vi "Periodic Tasks.vi"(8 "error in":errorcluster) -> ()   [LabVIEW 2019]
doc: "This VI runs in parallel to other tasks. It can contain as many user-defined periodic loops as you need. These can carry out PID or other sorts of timed response."
uses:
  <vilib>/Rock Robotics/WPI/Utilities/WPI_GetSetVariantRefNum.vi
  Robot Global Data.vi
  Secret_Control_Library_Protected/TIME_GET.vi
  <vilib>/addons/control/pid/pid.llb/PID (DBL).vi
  <vilib>/Rock Robotics/Network Tables/NT Write Numeric Array.vi
  <vilib>/Rock Robotics/Network Tables/NT Write Number.vi
  <vilib>/Rock Robotics/Network Tables/NT Write Boolean.vi
  Secret_Control_Library_Protected/Secret_Control_Library_Protected.lvlib
  <vilib>/addons/control/pid/NI_PID_pid.lvlib
  <vilib>/Rock Robotics/WPI/ThirdParty/JAS_Junk/TrajLib/Trajectory_Library.lvlib
panel:
  in  "Speed PID":T1={"proportional gain (Kc)"=0.6, "integral time (Ti, min)"=0.015, "derivative time (Td, min)"=0.0} {"derivative time (Td, min)" format="%.3f"; "integral time (Ti, min)" format="%.3f"; "proportional gain (Kc)" format="%.3f"}
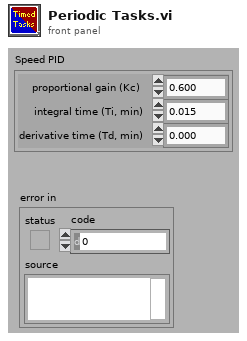
[diagram p1: front panel]
types:
  T1 = cluster{"proportional gain (Kc)":dbl, "integral time (Ti, min)":dbl, "derivative time (Td, min)":dbl}
  T2 = typedef "WPI_EncoderDevRef.ctl" = cluster{"DevStatus":errorcluster, "EncoderIndex":T3, "CounterIndex":T4, "DistancePerCount":dbl, "Decoding Type":T5}
  T3 = typedef "FPGA_EncoderIdx.ctl" = enum8{"Enc 0", "Enc 1", "Enc 2", "Enc 3", "Enc 4", "Enc 5", "Enc 6", "Enc 7", "Invalid"}
  T4 = typedef "FPGA_CounterCtrSystemIndex.ctl" = enum8{"Ctr 0", "Ctr 1", "Ctr 2", "Ctr 3", "Ctr 4", "Ctr 5", "Ctr 6", "Ctr 7", "Invalid"}
  T5 = typedef "WPI_EncoderType.ctl" = enum16{"1x", "2x", "4x"}
  T6 = typedef "WPI_GyroDevRef.ctl" = cluster{"DevStatus":errorcluster, "Analog Channel":T7, "Gain (VoltsPerDegree/Second)":dbl, "Gyro Type":enum16{"Analog", "XRS450"}, "Handle":i32, "SPI Bus":T8, "Device Found":bool, "Sample Rate":dbl, "Calibrate On Open":bool, "Offset":dbl}
  T7 = typedef "FPGA_AIChannel.ctl" = enum8{"AI 0", "AI 1", "AI 2", "AI 3", "AI MXP 0", "AI MXP 1", "AI MXP 2", "AI MXP 3", "Invalid"}
  T8 = typedef "spi_bus.ctl" = enum16{"SPI On-Board, CS0", "SPI On-Board, CS1", "SPI On-Board, CS2", "SPI On-Board, CS3", "SPI MXP", "Invalid"}
  T9 = typedef "WPI_RobotDriveDevRef.ctl" = cluster{"DevStatus":errorcluster, "Motors[]":T10[], "Square Inputs":bool, "Max Output":dbl}
  T10 = typedef "WPI_MotorControlDeviceRef.ctl" = cluster{"DeviceStatus":errorcluster, "Type":T11, "PWM":cluster{"PWM Channel":T12, "DeadBand":T13}, "CAN":cluster{"Device Number":u8, "SetOutput VI Ref":variant, "GetOutput VI Ref":variant, "Enable VI Ref":variant, "Disable VI Ref":variant, "Data":variant}, "Invert":bool, "DIO PWM":cluster{"PWM \"Enable\" Channel":T12, "DIOChannel":T14, "PWM Rate":dbl}}
  T11 = typedef "WPI_MotorControlType.ctl" = enum16{"PWM", "CAN", "DIO PWM"}
  T12 = typedef "FPGA_DIOPWMChannel.ctl" = enum8{"PWM 0", "PWM 1", "PWM 2", "PWM 3", "PWM 4", "PWM 5", "PWM 6", "PWM 7", "PWM 8", "PWM 9", "PWM MXP 0", "PWM MXP 1", "PWM MXP 2", "PWM MXP 3", "PWM MXP 4", "PWM MXP 5", "PWM MXP 6", "PWM MXP 7", "PWM MXP 8", "PWM MXP 9", "Invalid"}
  T13 = typedef "WPI_PWMDeadband.ctl" = cluster{"Name":string, "maxPositivePwm":i32, "minPositivePwm":i32, "centerPwm":i32, "maxNegativePwm":i32, "minNegativePwm":i32, "angularRange":u16}
  T14 = typedef "FPGA_DIOChannel.ctl" = enum8{"DIO 0", "DIO 1", "DIO 2", "DIO 3", "DIO 4", "DIO 5", "DIO 6", "DIO 7", "DIO 8", "DIO 9", "DIO MXP 0", "DIO MXP 1", "DIO MXP 2", "DIO MXP 3", "DIO MXP 4", "DIO MXP 5", "DIO MXP 6", "DIO MXP 7", "DIO MXP 8", "DIO MXP 9", "DIO MXP 10", "DIO MXP 11", "DIO MXP 12", "DIO MXP 13", "DIO MXP 14", "DIO MXP 15", "SPI Port CS1", "SPI Port CS2", "SPI Port CS3", "SPI Port MISO", "SPI Port MOSI", "Invalid"}
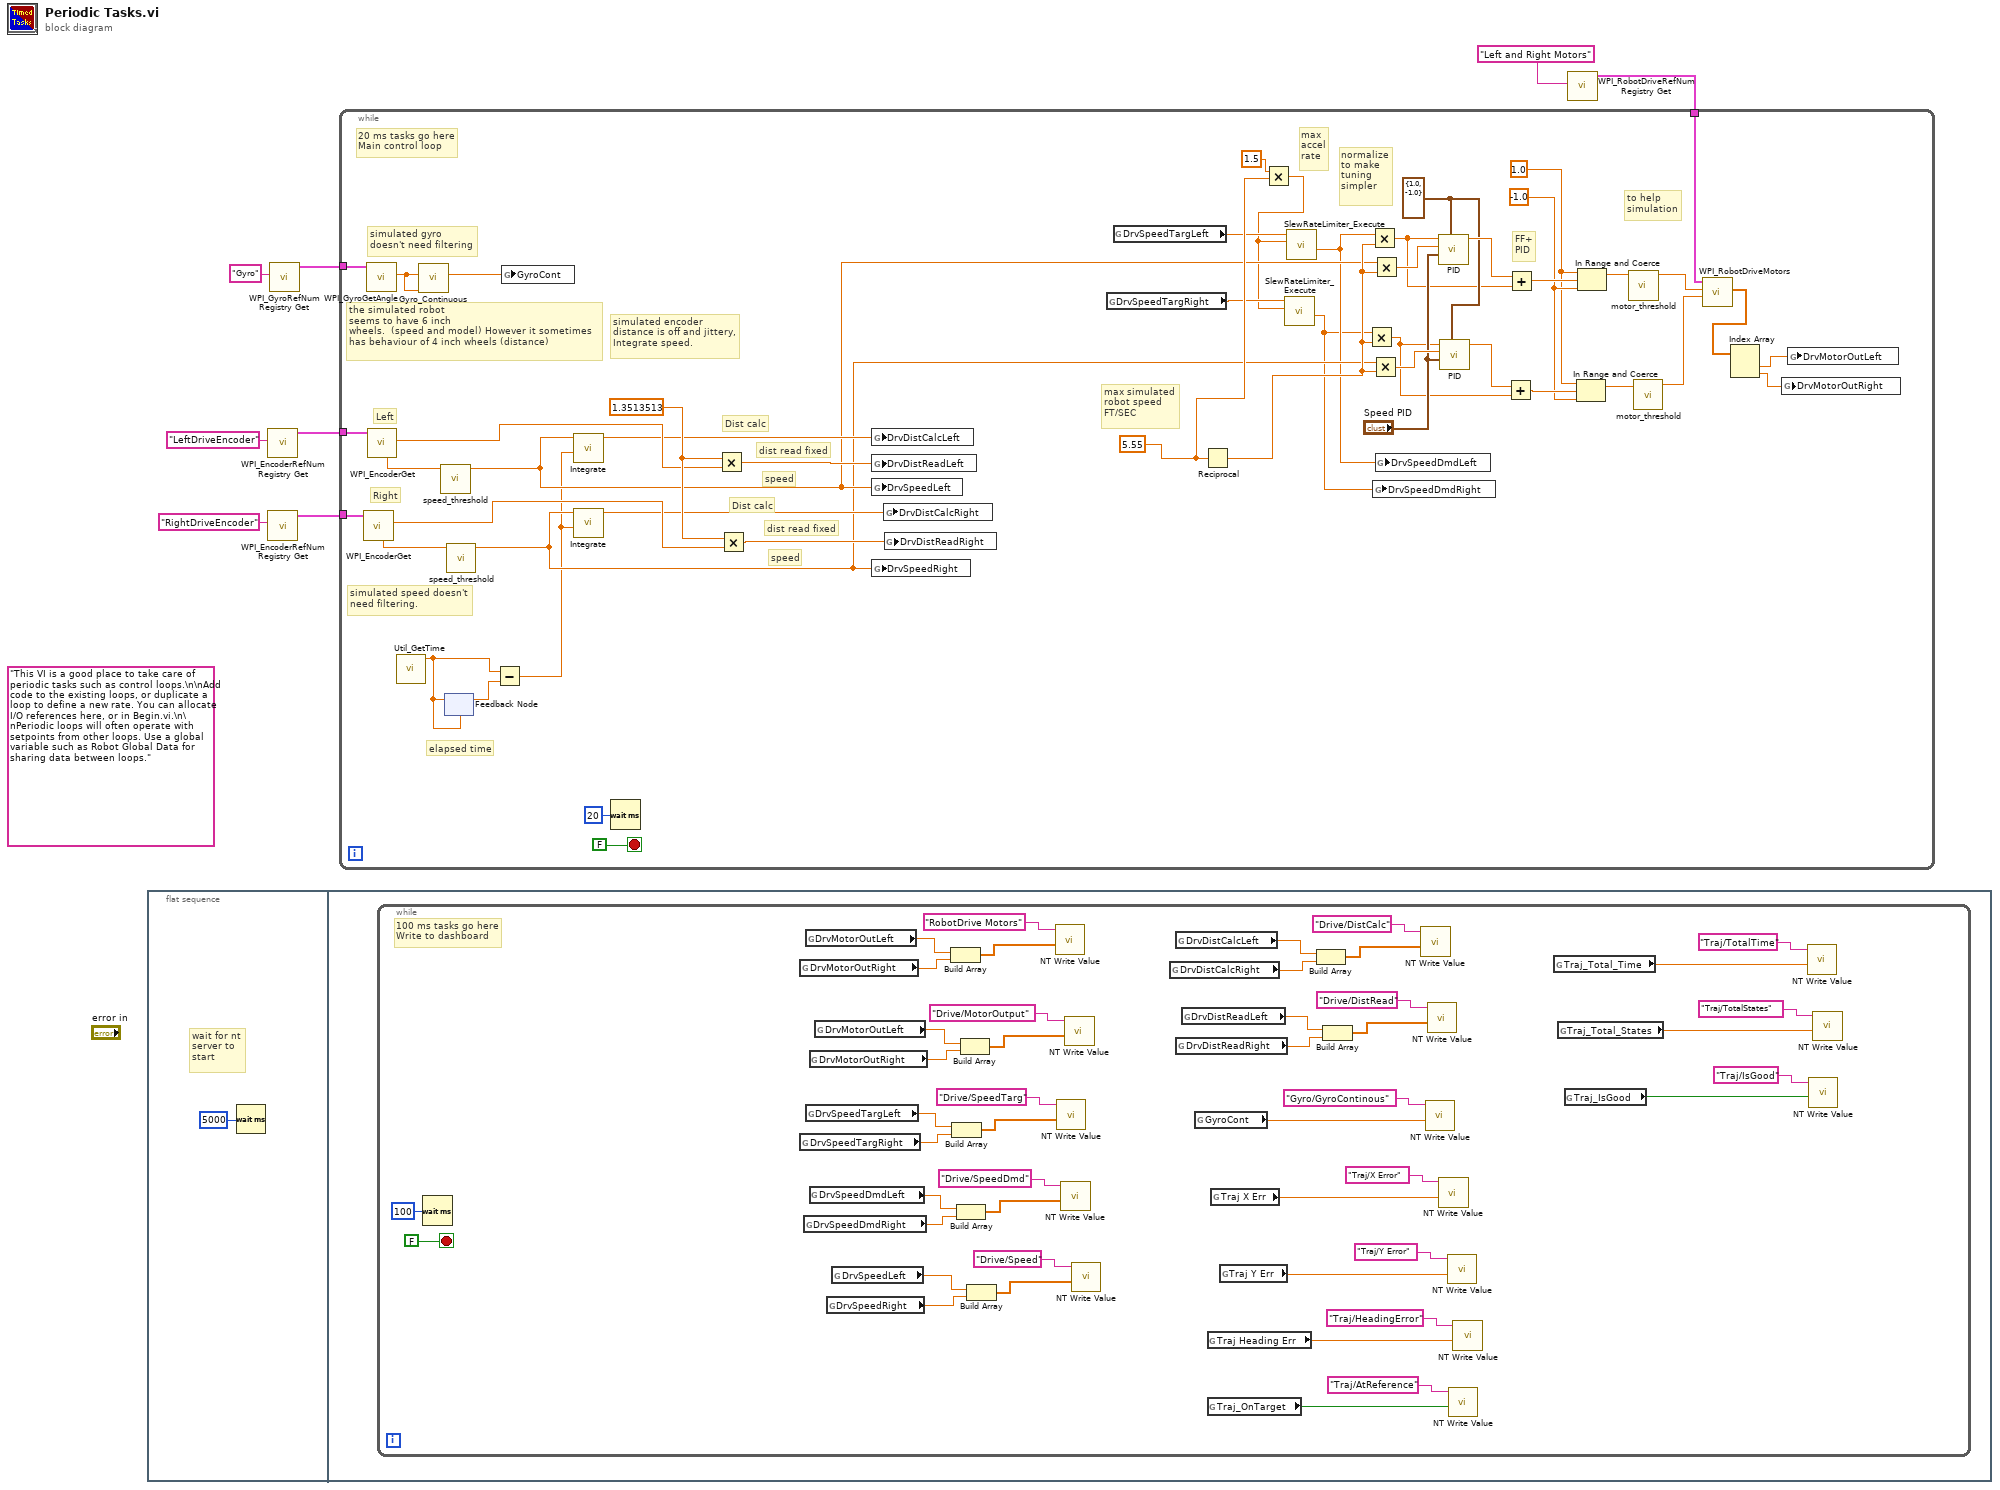
[diagram p0: block diagram]
diagram:
  (unwired) "This VI is a good place to take care of periodic tasks such as control loops.\n\nAdd code to the existing loops, or duplicate a loop to define a new rate. You can allocate I/O references here, or in Begin.vi.\n\nPeriodic loops will often operate with setpoints from other loops. Use a global variable such as Robot Global Data for sharing data between loops."
  n1 = flat-sequence {
    frame #0 {
      # "wait for nt\nserver to \nstart"
      n2 = Wait (ms)(milliseconds to wait=u32 5000) -> ()  [unwired: 1 out]
    }
    frame #1 {
      n3 = while {
        stop <- FALSE stop-if-true
        # "100 ms tasks go here\nWrite to dashboard"
        n4 = Wait (ms)(milliseconds to wait=u32 100) -> ()  [unwired: 1 out]
        n5 = global read "Robot Global Data.vi" "DrvMotorOutRight"() -> (w52:dbl)
        n6 = global read "Robot Global Data.vi" "DrvSpeedTargRight"() -> (w44:dbl)
        n7 = global read "Robot Global Data.vi" "DrvSpeedDmdRight"() -> (w40:dbl)
        n8 = global read "Robot Global Data.vi" "DrvMotorOutLeft"() -> (w53:dbl)
        n9 = global read "Robot Global Data.vi" "DrvSpeedTargLeft"() -> (w45:dbl)
        n10 = global read "Robot Global Data.vi" "DrvMotorOutRight"() -> (w48:dbl)
        n11 = global read "Robot Global Data.vi" "DrvSpeedDmdLeft"() -> (w41:dbl)
        n12 = global read "Robot Global Data.vi" "DrvMotorOutLeft"() -> (w49:dbl)
        n13 = global read "Robot Global Data.vi" "DrvSpeedRight"() -> (w36:dbl)
        n14 = global read "Robot Global Data.vi" "DrvSpeedLeft"() -> (w37:dbl)
        n15 = Build Array(w53, w52) -> (w51:dbl[])
        n16 = Build Array(w45, w44) -> (w43:dbl[])
        n17 = Build Array(w41, w40) -> (w39:dbl[])
        n18 = Build Array(w49, w48) -> (w47:dbl[])
        n19 = Build Array(w37, w36) -> (w35:dbl[])
        n20 = call-poly <vilib>:"NT Write Value.vi"("Numeric Array"=w51, "Name"="RobotDrive Motors") -> ()  [unwired: 9 in, 1 out]
        n21 = call-poly <vilib>:"NT Write Value.vi"("Numeric Array"=w43, "Name"="Drive/SpeedTarg") -> ()  [unwired: 9 in, 1 out]
        n22 = call-poly <vilib>:"NT Write Value.vi"("Numeric Array"=w39, "Name"="Drive/SpeedDmd") -> ()  [unwired: 9 in, 1 out]
        n23 = call-poly <vilib>:"NT Write Value.vi"("Numeric Array"=w47, "Name"="Drive/MotorOutput") -> ()  [unwired: 9 in, 1 out]
        n24 = call-poly <vilib>:"NT Write Value.vi"("Numeric Array"=w35, "Name"="Drive/Speed") -> ()  [unwired: 9 in, 1 out]
        n25 = global read "Robot Global Data.vi" "DrvDistCalcRight"() -> (w32:dbl)
        n26 = global read "Robot Global Data.vi" "DrvDistCalcLeft"() -> (w33:dbl)
        n27 = global read "Robot Global Data.vi" "DrvDistReadRight"() -> (w28:dbl)
        n28 = global read "Robot Global Data.vi" "DrvDistReadLeft"() -> (w29:dbl)
        n29 = global read "Robot Global Data.vi" "GyroCont"() -> (w24:dbl)
        n30 = global read "Robot Global Data.vi" "Traj Heading Err"() -> (w18:dbl)
        n31 = global read "Robot Global Data.vi" "Traj_OnTarget"() -> (w16:bool)
        n32 = global read "Robot Global Data.vi" "Traj X Err"() -> (w22:dbl)
        n33 = global read "Robot Global Data.vi" "Traj Y Err"() -> (w20:dbl)
        n34 = Build Array(w33, w32) -> (w31:dbl[])
        n35 = Build Array(w29, w28) -> (w27:dbl[])
        n36 = call-poly <vilib>:"NT Write Value.vi"("Numeric Array"=w31, "Name"="Drive/DistCalc") -> ()  [unwired: 9 in, 1 out]
        n37 = call-poly <vilib>:"NT Write Value.vi"("Numeric"=w24, "Name"="Gyro/GyroContinous") -> ()  [unwired: 9 in, 1 out]
        n38 = call-poly <vilib>:"NT Write Value.vi"("Numeric Array"=w27, "Name"="Drive/DistRead") -> ()  [unwired: 9 in, 1 out]
        n39 = call-poly <vilib>:"NT Write Value.vi"("Numeric"=w22, "Name"="Traj/X Error") -> ()  [unwired: 9 in, 1 out]
        n40 = call-poly <vilib>:"NT Write Value.vi"("Numeric"=w20, "Name"="Traj/Y Error") -> ()  [unwired: 9 in, 1 out]
        n41 = call-poly <vilib>:"NT Write Value.vi"("Boolean"=w16, "Name"="Traj/AtReference") -> ()  [unwired: 9 in, 1 out]
        n42 = call-poly <vilib>:"NT Write Value.vi"("Numeric"=w18, "Name"="Traj/HeadingError") -> ()  [unwired: 9 in, 1 out]
        n43 = global read "Robot Global Data.vi" "Traj_Total_Time"() -> (w12:dbl)
        n44 = global read "Robot Global Data.vi" "Traj_Total_States"() -> (w11:dbl)
        n45 = global read "Robot Global Data.vi" "Traj_IsGood"() -> (w10:bool)
        n46 = call-poly <vilib>:"NT Write Value.vi"("Numeric"=w12, "Name"="Traj/TotalTime") -> ()  [unwired: 9 in, 1 out]
        n47 = call-poly <vilib>:"NT Write Value.vi"("Boolean"=w10, "Name"="Traj/IsGood") -> ()  [unwired: 9 in, 1 out]
        n48 = call-poly <vilib>:"NT Write Value.vi"("Numeric"=w11, "Name"="Traj/TotalStates") -> ()  [unwired: 9 in, 1 out]
      }
    }
  }
  n49 = call <vilib>:"WPI_EncoderRefNum Registry Get.vi"("refnum name"="LeftDriveEncoder") -> ("EncoderDevRef"=w6:T2)  [unwired: 9 in, 1 out]
  n50 = call <vilib>:"WPI_EncoderRefNum Registry Get.vi"("refnum name"="RightDriveEncoder") -> ("EncoderDevRef"=w7:T2)  [unwired: 9 in, 1 out]
  n51 = call <vilib>:"WPI_GyroRefNum Registry Get.vi"("refnum name"="Gyro") -> ("GyroDevRef"=w2:T6)  [unwired: 9 in, 1 out]
  n52 = call <vilib>:"WPI_RobotDriveRefNum Registry Get.vi"("refnum name"="Left and Right Motors") -> ("RobotDriveDevRef"=w1:T9)  [unwired: 1 in, 9 out]
  n53 = while {
    tunnel: w7 -> [w99]
    tunnel: w6 -> [w98]
    tunnel: w2 -> [w96]
    tunnel: w1 -> [w82]
    stop <- FALSE stop-if-true
    w73 = 5.55
    w91 = -1.0 ("lower limit")
    w90 = 1.0 ("upper limit")
    w88 = cluster{"output high":dbl, "output low":dbl} {"output high"=1.0, "output low"=-1.0} ("output range")
    w102 = 1.3513513
    # "elapsed time"
    # "to help\nsimulation"
    # "simulated speed doesn't\nneed filtering."
    # "max simulated\nrobot speed\nFT/SEC"
    # "max\naccel\nrate"
    # "normalize\nto make\ntuning\nsimpler"
    # "FF+\nPID"
    # "simulated gyro \ndoesn't need filtering"
    # "Right"
    # "Left"
    # "the simulated robot\nseems to have 6 inch\nwheels.  (speed and model) However it sometimes\nhas behaviour of 4 inch wheels (distance)"
    # "speed"
    # "dist read fixed"
    # "Dist calc"
    # "speed"
    # "dist read fixed"
    # "Dist calc"
    # "simulated encoder\ndistance is off and jittery,\nIntegrate speed."
    # "20 ms tasks go here\nMain control loop"
    n54 = call <vilib>:"WPI_EncoderGet.vi"("EncoderDevRef"=w99) -> ("Distance"=w100:dbl, "Rate"=w70:dbl)  [unwired: 5 in, 4 out]
    n55 = call <vilib>:"WPI_GyroGetAngle.vi"("GyroDevRef"=w96) -> ("Angle"=w97:dbl)  [unwired: 7 in, 3 out]
    n56 = call <vilib>:"WPI_EncoderGet.vi"("EncoderDevRef"=w98) -> ("Distance"=w101:dbl, "Rate"=w72:dbl)  [unwired: 5 in, 4 out]
    n57 = call <vilib>:"Util_GetTime.vi"() -> ("FPGA_Time_Seconds"=w62:dbl)  [unwired: 9 in, 2 out]
    n58 = call "Gyro_Continuous.vi"("GyroInitial"=w97, "GyroInput"=w97) -> ("GyroContinuous"=w64:dbl)  [unwired: 9 in]
    n59 = call "speed_threshold.vi"("SPEED IN"=w72) -> ("SPEED OUT"=w71:dbl)  [unwired: 10 in]
    n60 = feedback-in #1(w62) -> ()
    n61 = feedback #1(w62) -> (w63:dbl)
    n62 = call "speed_threshold.vi"("SPEED IN"=w70) -> ("SPEED OUT"=w69:dbl)  [unwired: 10 in]
    n63 = Subtract(x=w62, y=w63) -> (x-y=w61:dbl)
    n64 = global write "Robot Global Data.vi" "GyroCont"(w64) -> ()
    n65 = call "Integrate.vi"("Elapsed Sec"=w61, "Rate"=w71) -> ("DIST"=w81:dbl)  [unwired: 9 in]
    n66 = call "Integrate.vi"("Elapsed Sec"=w61, "Rate"=w69) -> ("DIST"=w79:dbl)  [unwired: 9 in]
    n67 = Wait (ms)(milliseconds to wait=u32 20) -> ()  [unwired: 1 out]
    n68 = Multiply(x=w102, y=w101) -> (x*y=w80:dbl)
    n69 = Multiply(x=w102, y=w100) -> (x*y=w78:dbl)
    n70 = global write "Robot Global Data.vi" "DrvDistCalcLeft"(w81) -> ()
    n71 = global write "Robot Global Data.vi" "DrvDistReadLeft"(w80) -> ()
    n72 = global write "Robot Global Data.vi" "DrvSpeedLeft"(w71) -> ()
    n73 = global write "Robot Global Data.vi" "DrvSpeedRight"(w69) -> ()
    n74 = global write "Robot Global Data.vi" "DrvDistCalcRight"(w79) -> ()
    n75 = global write "Robot Global Data.vi" "DrvDistReadRight"(w78) -> ()
    n76 = global read "Robot Global Data.vi" "DrvSpeedTargRight"() -> (w57:dbl)
    n77 = global read "Robot Global Data.vi" "DrvSpeedTargLeft"() -> (w59:dbl)
    n78 = Reciprocal(x=w73) -> (1/x=w74:dbl)
    n79 = Multiply(x=1.5, y=w73) -> (x*y=w56:dbl)
    n80 = call <vilib>:"SlewRateLimiter_Execute.vi"("Rate"=w56, "Input"=w57) -> ("Output"=w58:dbl)  [unwired: 8 in, 1 out]
    n81 = call <vilib>:"SlewRateLimiter_Execute.vi"("Rate"=w56, "Input"=w59) -> ("Output"=w60:dbl)  [unwired: 8 in, 1 out]
    n82 = Multiply(x=w58, y=w74) -> (x*y=w85:dbl)
    n83 = Multiply(x=w60, y=w74) -> (x*y=w84:dbl)
    n84 = Multiply(x=w69, y=w74) -> (x*y=w89:dbl)
    n85 = Multiply(x=w71, y=w74) -> (x*y=w86:dbl)
    n86 = global write "Robot Global Data.vi" "DrvSpeedDmdRight"(w58) -> ()
    n87 = global write "Robot Global Data.vi" "DrvSpeedDmdLeft"(w60) -> ()
    n88 = call-poly <vilib>:"PID.vi"("output range"=w88, "PID gains"="Speed PID", "process variable"=w86, "setpoint"=w84) -> ("output"=w95:dbl)  [unwired: 6 in, 1 out]
    n89 = call-poly <vilib>:"PID.vi"("output range"=w88, "PID gains"="Speed PID", "process variable"=w89, "setpoint"=w85) -> ("output"=w93:dbl)  [unwired: 6 in, 1 out]
    n90 = Add(x=w93, y=w85) -> (x+y=w92:dbl)
    n91 = Add(x=w95, y=w84) -> (x+y=w94:dbl)
    n92 = In Range and Coerce(upper limit=w90, x=w92, lower limit=w91) -> (coerced(x)=w66:dbl)  [unwired: 1 out]
    n93 = In Range and Coerce(upper limit=w90, x=w94, lower limit=w91) -> (coerced(x)=w67:dbl)  [unwired: 1 out]
    n94 = call "motor_threshold.vi"("motor in"=w67) -> ("motor out"=w68:dbl)  [unwired: 10 in]
    n95 = call "motor_threshold.vi"("motor in"=w66) -> ("motor out"=w65:dbl)  [unwired: 10 in]
    n96 = call <vilib>:"WPI_RobotDriveMotors.vi"("RightSpeed"=w65, "LeftSpeed"=w68, "RobotDriveDevRef"=w82) -> ("Motor Values"=w77:dbl[])  [unwired: 6 in, 2 out]
    n97 = Index Array(array=w77) -> (element #1=w76:dbl, element #2=w75:dbl)  [unwired: 2 in]
    n98 = global write "Robot Global Data.vi" "DrvMotorOutRight"(w75) -> ()
    n99 = global write "Robot Global Data.vi" "DrvMotorOutLeft"(w76) -> ()
  }
